vi "Flattened Cluster to Flattened Elements.vi"(10 "Flattened Cluster":string, 11 "Cluster Type Descriptor":i16[](array[numeric])) -> (2 "Flattened Cluster Elements":string[](array[string]), 3 "Elements Type Descriptor":cluster{"Type Descriptor":i16[]}[](array[cluster]) {"Type Descriptor" format="%x"})   [LabVIEW 2020, in "OpenConvert.lvlib"]
uses:
  OpenConvert.lvlib
  _built_ppls/OpenDescriptor.lvlibp
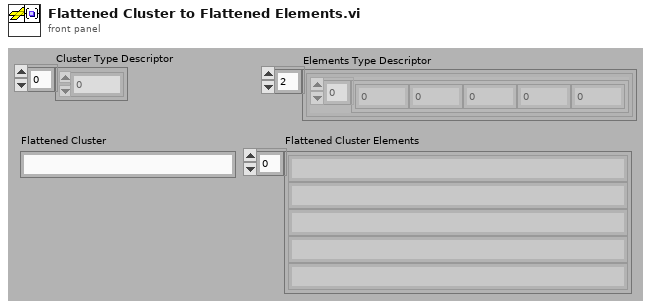
[diagram p1: front panel]
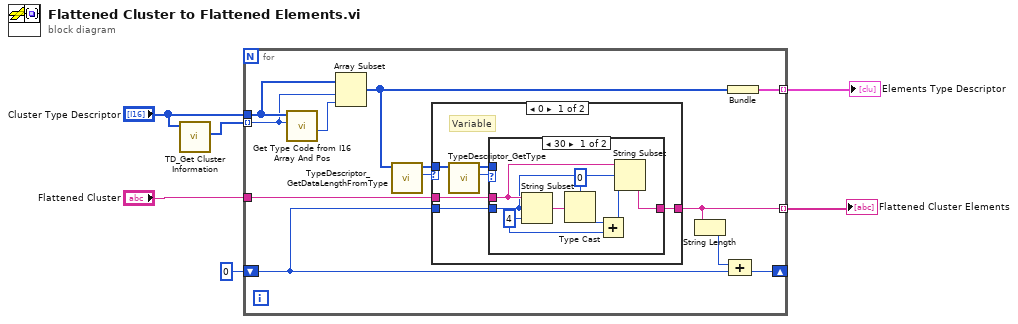
[diagram p0: block diagram]
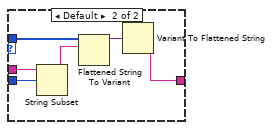
[diagram p2: hidden frame]
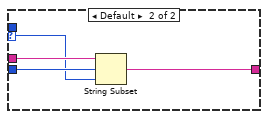
[diagram p3: hidden frame]
diagram:
  n1 = call <vilib>:"TD_Get Cluster Information.vi"("Type descriptor"="Cluster Type Descriptor") -> ("Contained TD Offsets"=w6:i32[])  [unwired: 9 in, 1 out]
  n2 = for {
    tunnel: w6 -> [w17] mode=indexing
    tunnel: "Cluster Type Descriptor" -> [w18]
    tunnel: [w15] -> w5 mode=indexing
    tunnel: "Flattened Cluster" -> [w12]
    tunnel: [w9] -> w3 mode=indexing
    shift-right: [w11] -> _
    shift-left: 0 -> [w13]
    n3 = call <vilib>:"Get Type Code from I16 Array And Pos.vi"("Pos in Type Descriptor (0)"=w17, "Type descriptor"=w18) -> ("Size (Words)"=w16:i32)  [unwired: 7 in, 2 out]
    n4 = Array Subset(array=w18, index=w17, length=w16) -> (w7:i16[])
    n5 = call "TypeDescriptor_GetDataLengthFromType.vi"("type descriptor"=w7) -> ("Length"=w10:u32, "type descriptor dup"=w8:i16[])  [unwired: 9 in]
    n6 = case shown="0" w10 {
      selector: w10 -> [_ w39]
      tunnel: w13 -> [w22 w42]
      tunnel: w12 -> [w23 w41]
      tunnel: [w24 w40] -> w9
      tunnel: w8 -> [w21 _]
      frame 0 {
        # "Variable"
        n7 = call "TypeDescriptor_GetType.vi"("type descriptor"=w21) -> ("Type"=w19:u8, "type descriptor dup"=w20:i16[])  [unwired: 9 in]
        n8 = case shown="30" w19 {
          tunnel: [w30 w37] -> w24
          tunnel: w23 -> [w29 w36]
          tunnel: w22 -> [w28 w35]
          tunnel: w20 -> [_ w33]
          frame 48 {
            w26 = 4 ("length (rest)")
            n9 = String Subset(string=w29, offset (0)=w28, length (rest)=w26) -> (substring=w31:string)
            n10 = Type Cast(type=u32 0, x=w31) -> (*(type *) &x=w27:u32)
            n11 = Add(x=w27, y=w26) -> (x+y=w25:u32)
            n12 = String Subset(string=w29, offset (0)=w28, length (rest)=w25) -> (substring=w30:string)
          }
          frame Default {
            n13 = String Subset(string=w36, offset (0)=w35) -> (substring=w34:string)  [unwired: 1 in]
            n14 = Flattened String To Variant(6:w34, 7:w33) -> (3:w38:variant)  [unwired: 1 in, 1 out]
            n15 = Variant To Flattened String(Variant=w38) -> (data string=w37:string)  [unwired: 1 out]
          }
        }
      }
      frame Default {
        n16 = String Subset(string=w41, offset (0)=w42, length (rest)=w39) -> (substring=w40:string)
      }
    }
    n17 = String Length(string=w9) -> (length=w14:i32)
    n18 = Bundle(w7) -> (w15:cluster{i16[]})  [unwired: 1 in]
    n19 = Compound Arithmetic op=ADD(w14, w13) -> (w11:i32)
  }
  "Flattened Cluster Elements" <- w3
  "Elements Type Descriptor" <- w5
